vi "7961 FPGA.vi"() -> ()   [LabVIEW 2015]
uses:
  Controls/FPGA_Frame State.ctl
  <vilib>/Platform/TimedLoop/XDataNode/timing_clust.ctl
  <vilib>/Platform/TimedLoop/XDataNode/nitl_modes.ctl
  <vilib>/Platform/TimedLoop/XDataNode/wakeup.ctl
  <vilib>/rvi/FXPMathLib/FxpDiv/subVIs/nifxpmath_Div_SimConfig.ctl
  <vilib>/rvi/Emulation/niFpgaSctlEmulationGetInTimedLoop.vi
  <vilib>/rvi/Emulation/niFpgaProcessEmulError.vi
  <vilib>/rvi/Emulation/niFpgaEmulationReportErrorSimple.vi
  <vilib>/rvi/Emulation/niFpgaGetClockAttributes.vi
  <vilib>/rvi/Emulation/niFpgaCriticalErrorInLSC.vi
  <vilib>/rvi/eio/common/nirviEmuTemplateMethod_errors.vi
  <vilib>/rvi/interface/RandomDataEmulation/niFpgaRandomDataHandleErrors.vi
  <vilib>/rvi/Memory/Memory_Emulation/nirvimemoryFastEmulation.vi
  <vilib>/rvi/Memory/Memory_Emulation/nirvimemoryEmulation.vi
  <vilib>/rvi/Emulation/niFpgaEmulationIsFPGAContextNoSignature.vi
  <vilib>/rvi/DataTransferAndStorage/Container/Common/niFpgaContainerGetUniqueNameForEmu.vi
  <vilib>/rvi/errors/nirviReportUnexpectedCaseInternalError (U32).vi
  <vilib>/rvi/FXPMathLib/FxpDiv/simVIs/DllFxpDivTemp_sub.vi
  <vilib>/Platform/TimedLoop/XDataNode/XDataNode.xnode
  <vilib>/eio/EIONode/EIONode.xnode
  <vilib>/rvi/DataTransferAndStorage/Container/XNode/niFpgaContainer.xnode
  <vilib>/rvi/interface/RandomDataEmulation/nirviRandomDataFpgaReadWriteTemplate.vi
  <vilib>/rvi/FXPMathLib/FxpDiv/XNode/nifxpmath_Div.xnode
  <vilib>/Platform/TimedLoop/XDataNode/XDNodeRunTimeDep.lvlib
  <instrlib>/_niInstr/Basic Elements/v1/FPGA/niInstr Basic Elements v1 FPGA.lvlib
panel:
  in  "Remind":u32
  in  "Switch":bool
  in  "Point/Pixel":i16
  out "Ramp Number":u32
  out "Ramp 待读取元素数量":u32
  in  "Microscope":enum16{"Miniature", "Benchtop"}(ring)
  out "No Remind":bool
  out "Remind Element":u32
  in  "FOCUS":bool
  out "Wait Frame State":T1
  in  "Line":u16
  out "输出有效":bool
  out "运算溢出":bool
  in  "Pixel/Line":u16
  in  "Sanple Rate Divider":u16=1 min=1
  out "Adapter Module Present":bool
  out "Adapter Module ID Expected":u32
  out "Adapter Module ID Inserted":u32
  out "Adapter Module Initialization Done":bool
  out "Adapter Module ID Mismatch":bool
  in  "Adapter Module Do User Command Commit":bool caption="(Mech Action: Latch)"
  in  "Adapter Module User Command":u8
  out "Adapter Module User Command Idle":bool
  out "Adapter Module User Command Status":u8
  in  "Adapter Module User Data 0":u8
  in  "Adapter Module User Data 1":u8
  out "Adapter Module PLL Locked":bool
  # "Acquisition Parameters"
  # "Acquisition Control"
  # "User Command Load"
  # "Fpga status"
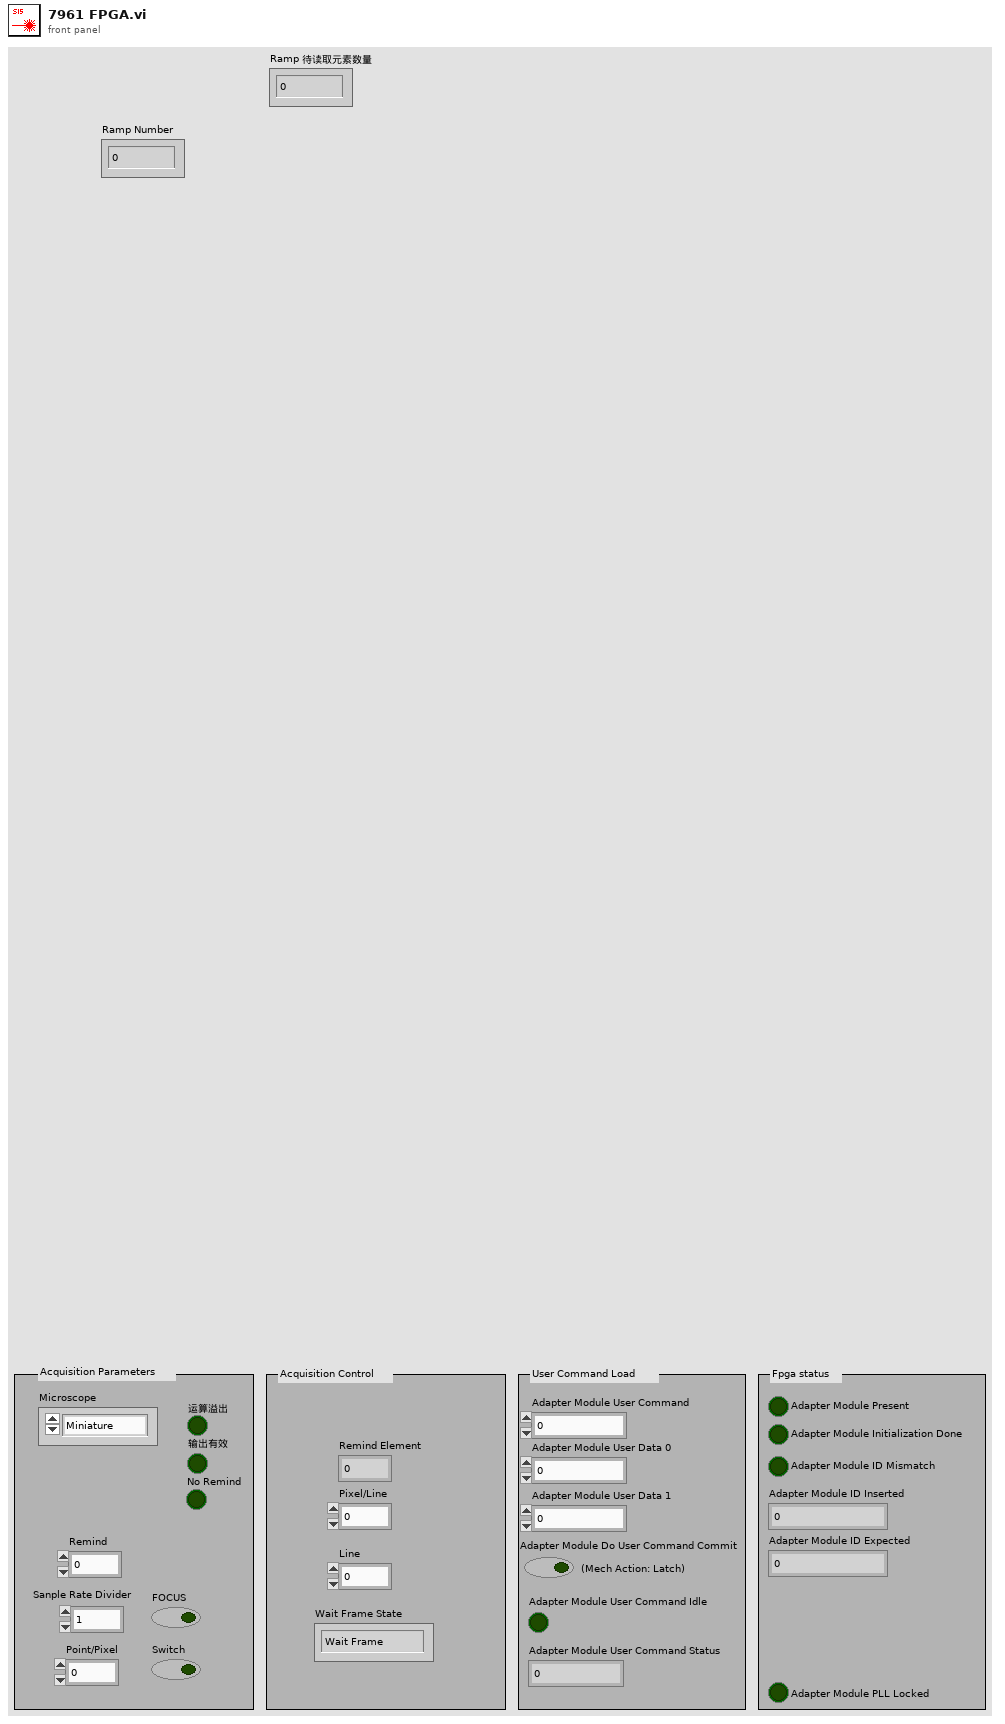
[diagram p1: front panel]
types:
  T1 = typedef "FPGA_Frame State.ctl" = enum16{"Wait Frame", "Start Frame", "Framing"}
  T2 = typedef "XDNodeRunTimeDep.lvlib/timing_clust.ctl" = cluster{"Expected End [f-1]":u64, "Actual End [f-1]":u64, "Finished Late? [f-1]":bool, "Expected End [i-1]":u64, "Actual End [i-1]":u64, "Finished Late? [i-1]":bool, "Expected Start [i]":u64, "Actual Start [i]":u64, "Expected Start [f]":u64, "Actual Start [f]":u64, "Source Name":string, "Structure Name":string, "Period":i64, "Deadline":i64, "Offset":i64, "Start":i64, "Priority":i32, "Timeout":i32, "Mode":T3, "Wakeup Reason":T4, "Error":errorcluster, "Source Type":string, "Secondary Source Type":string, "Global End Time":u64, "Global Start Time":u64, "Frame Duration":u64, "Iteration Duration":u64, "Assigned CPU":i32, "I/O Scan Engine Mode":u32}
  T3 = typedef "XDNodeRunTimeDep.lvlib/nitl_modes.ctl" = enum32{"No Change", "Process missed periods, maintain original phase", "Discard missed periods, maintain original phase", "Process missed periods, ignore original phase", "Discard missed periods, ignore original phase"}
  T4 = typedef "XDNodeRunTimeDep.lvlib/wakeup.ctl" = enum32{"Normal", "Aborted", "Asynchronous wakeup", "Timing source error", "Timed loop error", "Timeout"}
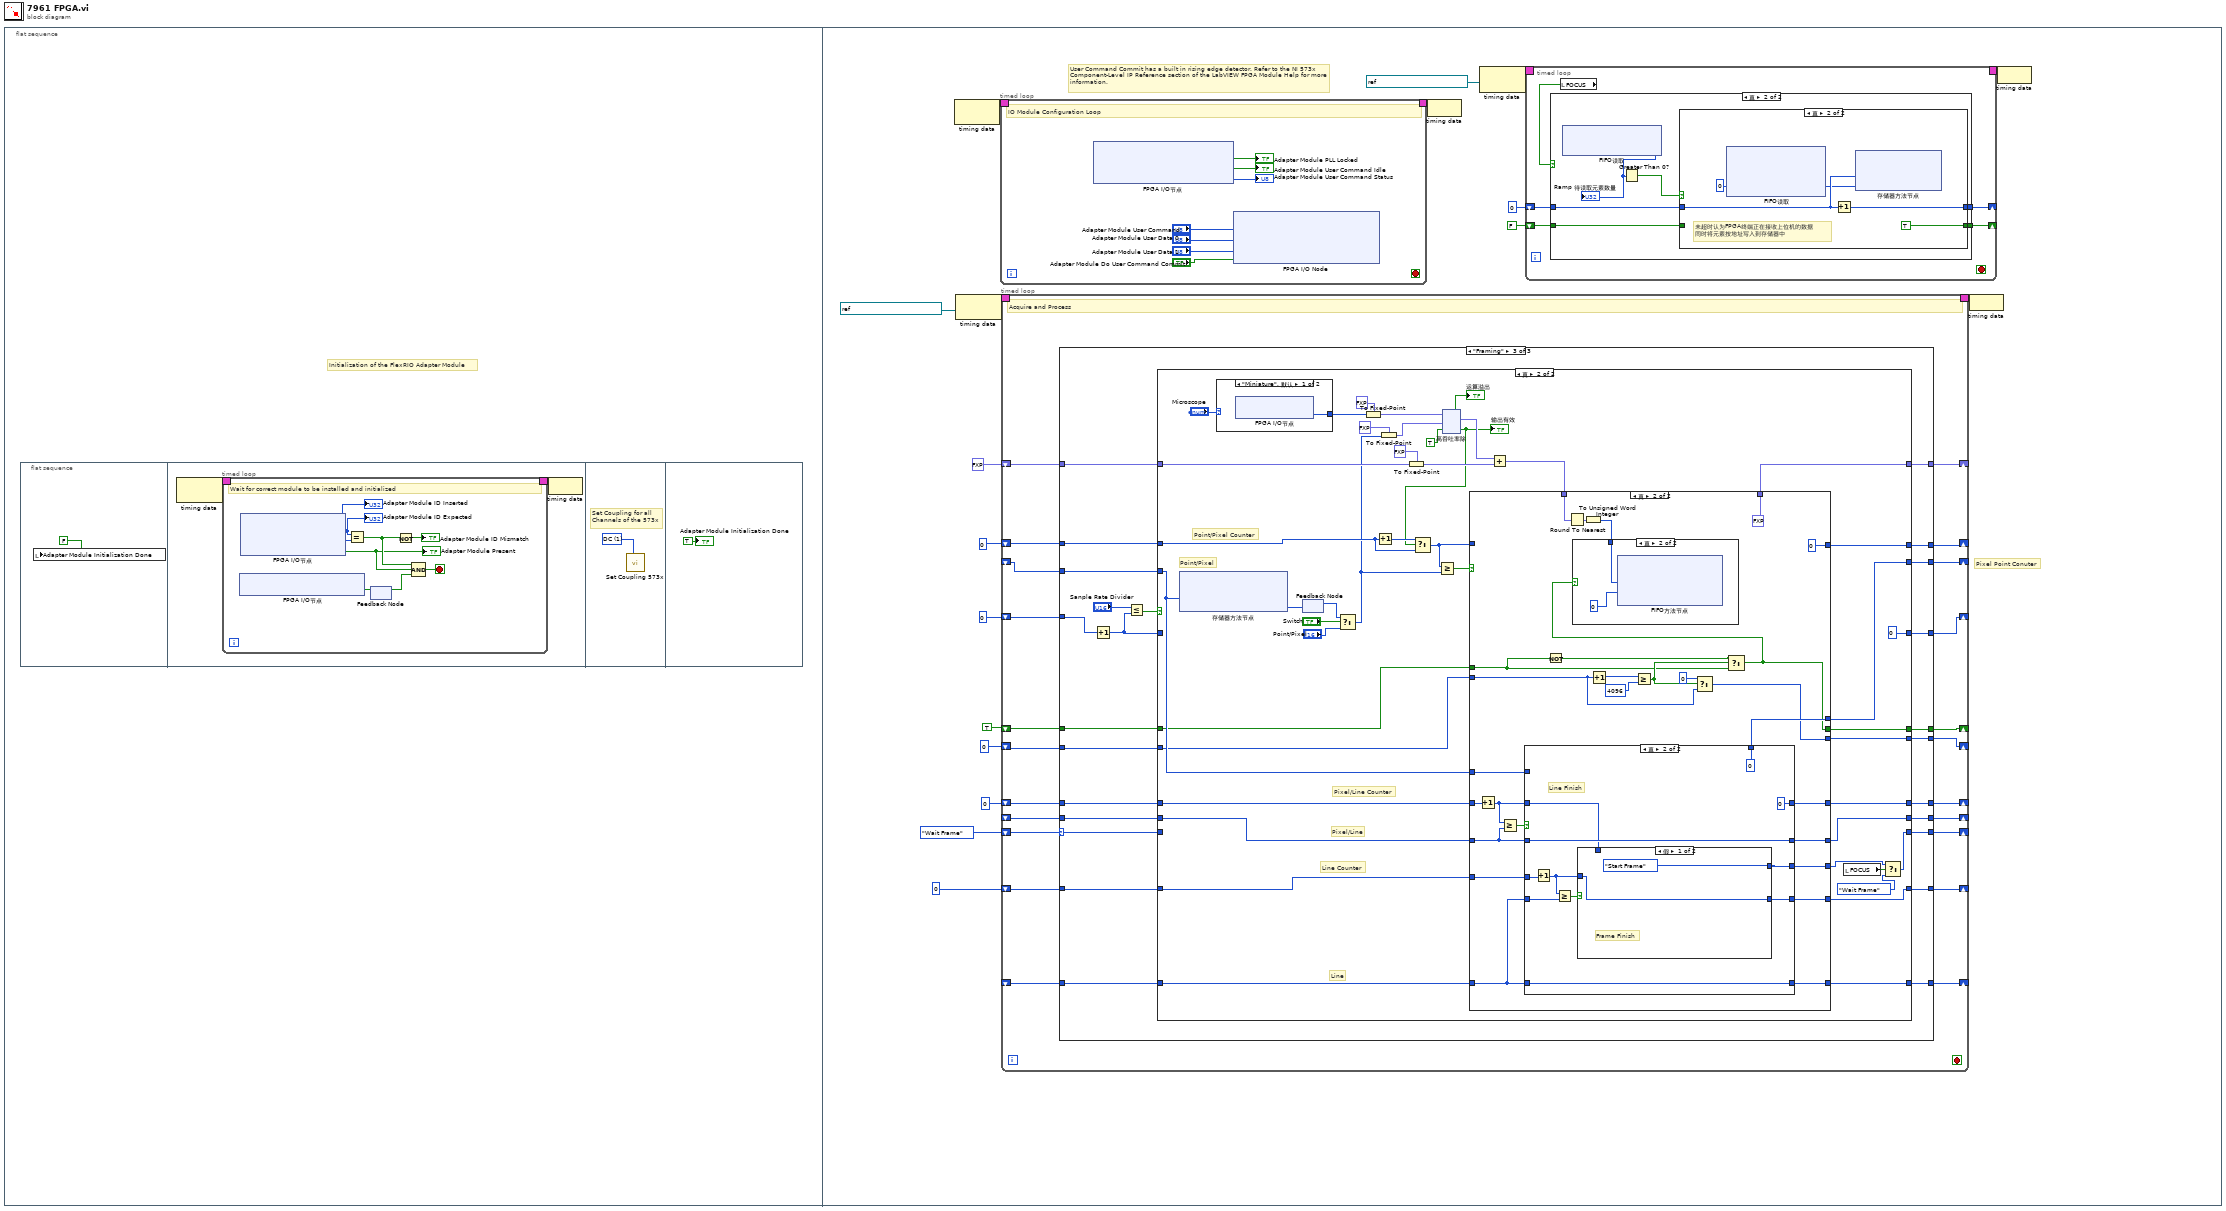
[diagram p0: block diagram]
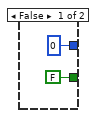
[diagram p2: hidden frame]
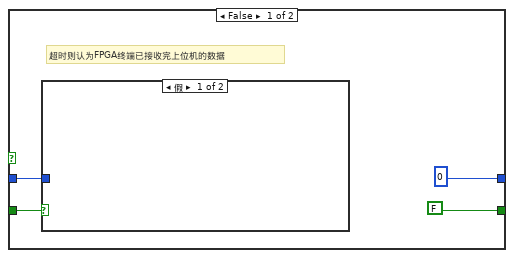
[diagram p3: hidden frame]
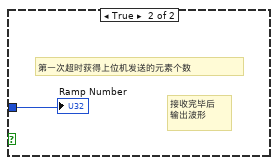
[diagram p4: hidden frame]
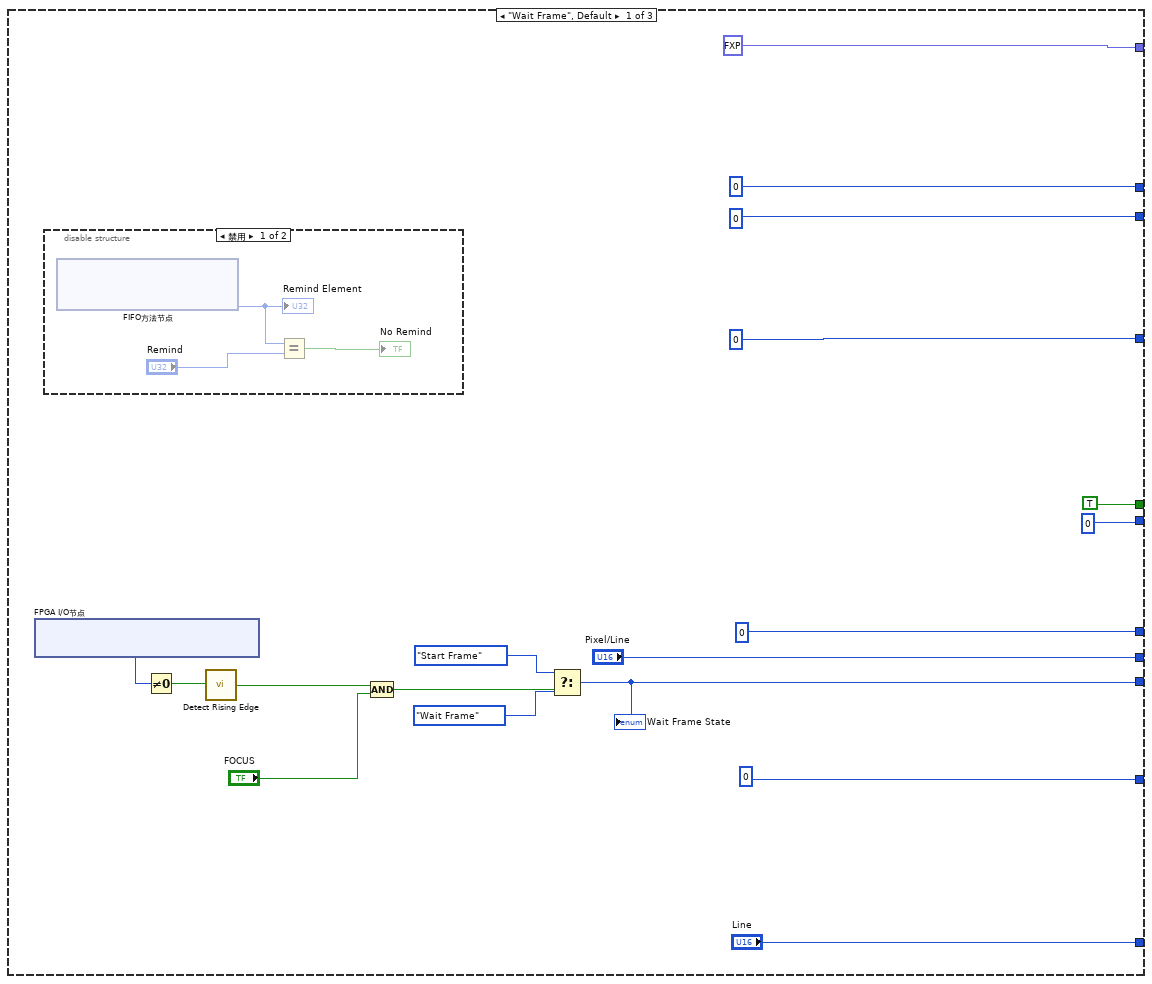
[diagram p5: hidden frame]
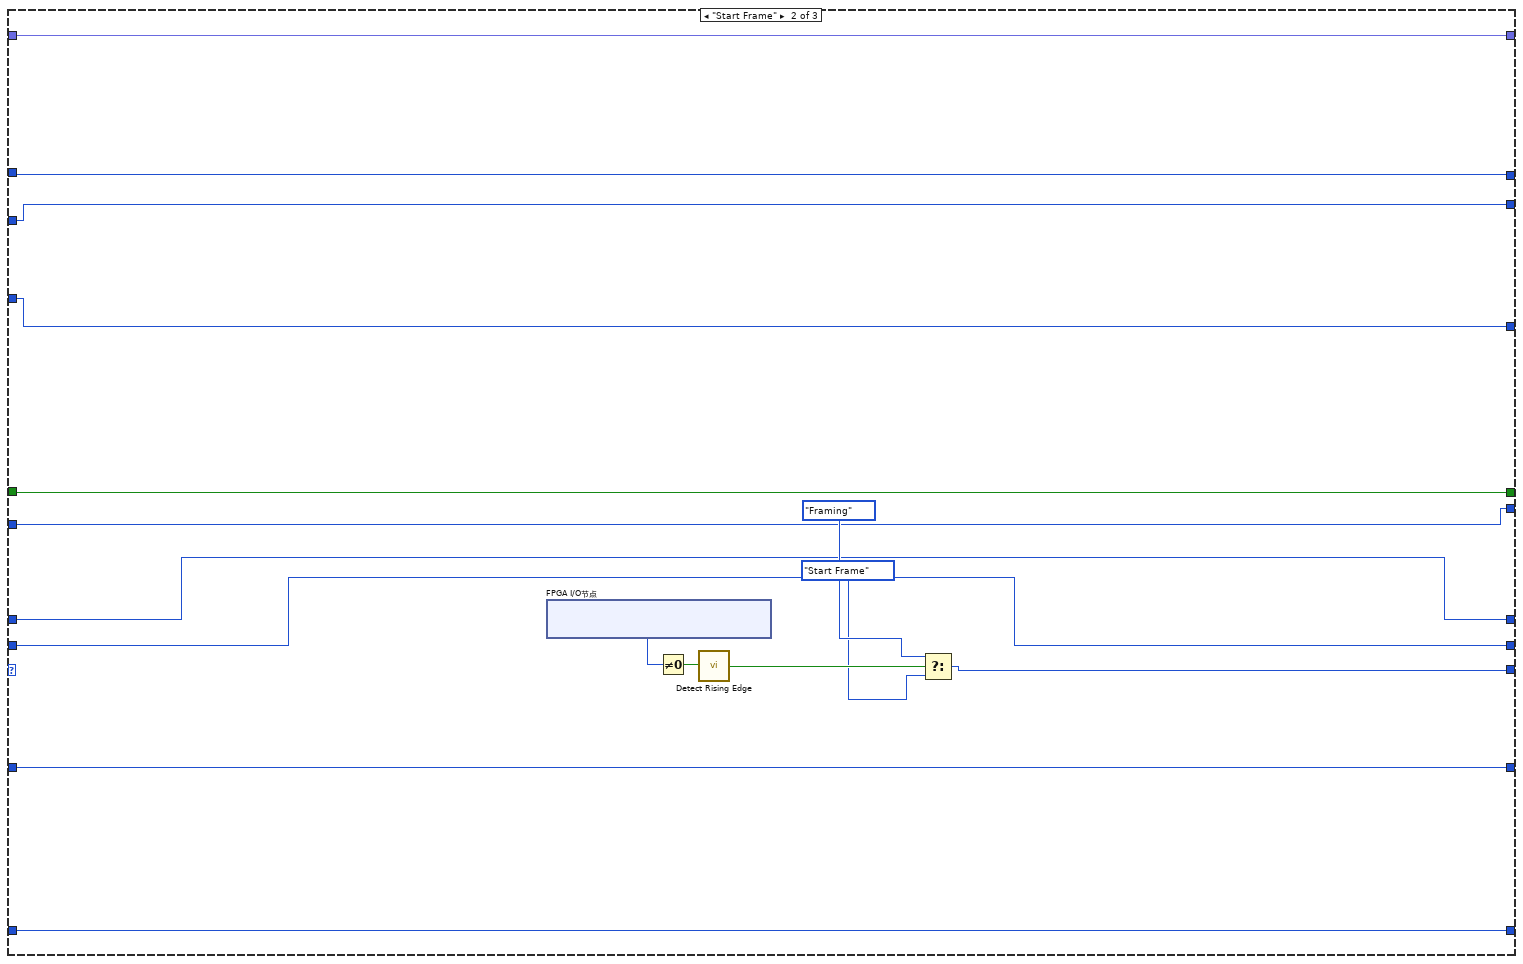
[diagram p7: hidden frame]
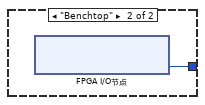
[diagram p9: hidden frame]
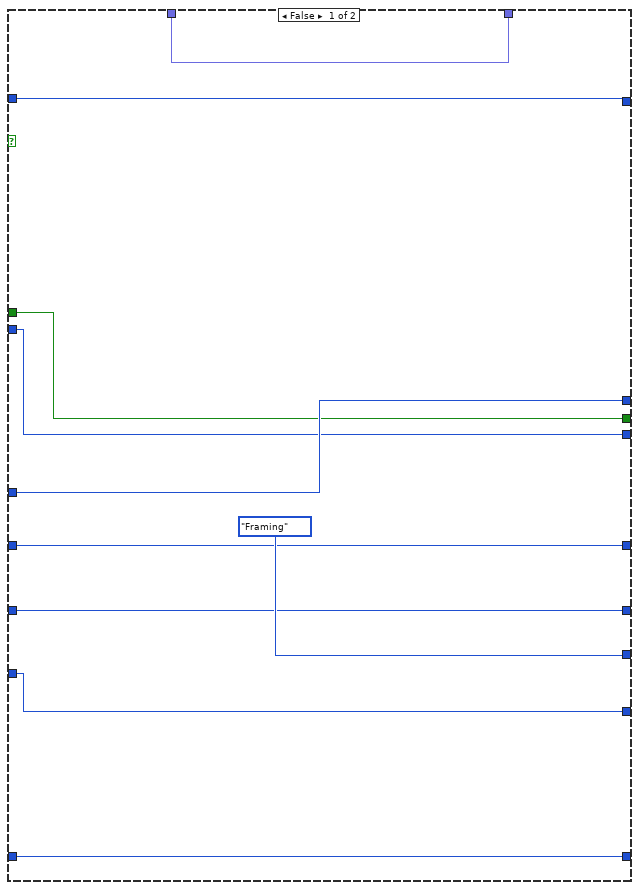
[diagram p10: hidden frame]
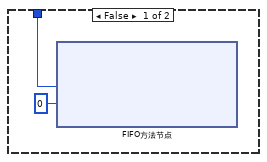
[diagram p11: hidden frame]
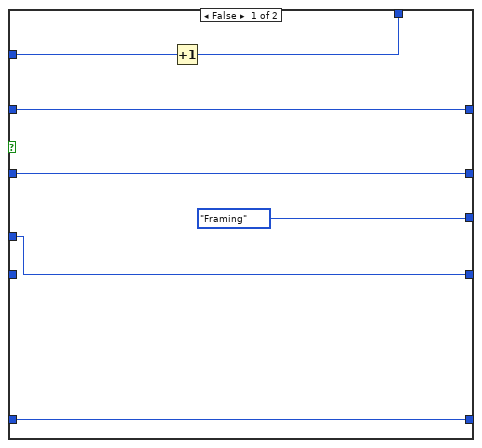
[diagram p12: hidden frame]
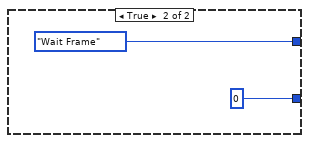
[diagram p13: hidden frame]
diagram:
  n1 = flat-sequence {
    frame #0 {
      # "Initialization of the FlexRIO Adapter Module"
      n2 = flat-sequence {
        frame #0 {
          n3 = local write "Adapter Module Initialization Done"(FALSE ("InitializationDone")) -> ()
        }
        frame #1 {
          n4 = node-c288() -> (w3:T2)  [unwired: 1 in]
          n5 = timed-loop {
            timing: w3 -> [_]
            timing-out: [_] -> w2
            stop <- w10 stop-if-true
            # "Wait for correct module to be installed and initialized"
            n6 = xnode "FPGA I/O节点"() -> ("IO Module\\Initialization Done"=w5:bool)  [unwired: 1 in, 1 out]
            n7 = xnode "FPGA I/O节点"() -> ("Expected IO Module ID"=w11:u32, "Inserted IO Module ID"=w9:u32, "IO Module Present"=w6:bool)  [unwired: 3 in, 3 out]
            "Adapter Module ID Inserted" <- w9
            "Adapter Module ID Expected" <- w11
            "Adapter Module Present" <- w6
            n8 = Equal?(x=w11, y=w9) -> (x = y?=w7:bool)
            n9 = feedback-in #1(w5) -> ()
            n10 = feedback #1() -> (w4:bool)  [unwired: 1 in]
            n11 = Not(x=w7) -> (.not. x?=→"Adapter Module ID Mismatch":bool)
            n12 = Compound Arithmetic op=AND(w7, w6, w4) -> (w10:bool)
          }
          n13 = node-c288(w2) -> ()
        }
        frame #2 {
          w16 = u8 1 items=["DC"=1, "AC"=0] ("Coupling")
          # "Set Coupling for all\nChannels of the 573x"
          n14 = call "Set Coupling 573x.vi"("Coupling"=w16) -> ()  [unwired: 11 in]
        }
        frame #3 {
          "Adapter Module Initialization Done" <- TRUE ("InitializationDone")
        }
      }
    }
    frame #1 {
      # "Pixel Point Conuter"
      # "User Command Commit has a built in rising edge detector. Refer to the NI 573x Component-Level IP Reference section of the LabVIEW FPGA Module Help for more information."
      n15 = node-c288() -> (w35:T2)  [unwired: 1 in]
      n16 = node-c288(refnum<k21> "IO Module\\Sample Clock" ("Source Name")) -> (w33:T2)
      n17 = timed-loop {
        timing: w35 -> [_]
        timing-out: [_] -> w34
        stop <- _ stop-if-true
        # "IO Module Configuration Loop"
        n18 = xnode "FPGA I/O节点"() -> ("IO Module\\PLL Locked"=→"Adapter Module PLL Locked":bool, "IO Module\\User Command Idle"=→"Adapter Module User Command Idle":bool, "IO Module\\User Command Status"=→"Adapter Module User Command Status":u8)  [unwired: 3 in, 3 out]
        n19 = xnode ("FPGA I/O Node")("IO Module\\User Command"="Adapter Module User Command", "IO Module\\User Data 0"="Adapter Module User Data 0", "IO Module\\User Data 1"="Adapter Module User Data 1", "IO Module\\User Command Commit"="Adapter Module Do User Command Commit") -> ()  [unwired: 4 in, 4 out]
      }
      n20 = timed-loop {
        timing: w33 -> [_]
        timing-out: [_] -> w32
        shift-right: [w85] -> _
        shift-left: u16 0 -> [w86]
        shift-right: [w83] -> _
        shift-left: FPGA_Frame_State."Wait Frame" ("Line State") -> [w84]
        shift-right: [w81] -> _
        shift-left: 0 ("t") -> [w82]
        shift-right: [w79] -> _
        shift-left: u16 0 ("t") -> [w80]
        shift-right: [w77] -> _
        shift-left: fxp<+,32,16> 0.0 ("x") -> [w78]
        shift-right: [w75] -> _
        shift-left: u16 0 ("t") -> [w76]
        shift-right: [w73] -> _
        shift-left: _ -> [w74]
        shift-right: [w71] -> _
        shift-left: _ -> [w72]
        shift-right: [w69] -> _
        shift-left: _ -> [w70]
        shift-right: [w67] -> _
        shift-left: TRUE ("x >= y?") -> [w68]
        shift-right: [w65] -> _
        shift-left: u16 0 -> [w66]
        stop <- _ stop-if-true
        # "Acquire and Process"
        n21 = case shown="\"Framing\"" w84 {
          selector: w84 -> [_ _ w146]
          tunnel: w86 -> [_ w112 w148]
          tunnel: [u16 0 w112 w147] -> w85
          tunnel: [w98 w119 w145] -> w83
          tunnel: w82 -> [_ w110 w141]
          tunnel: [0 ("t") w110 w140] -> w81
          tunnel: w80 -> [_ w113 w139]
          tunnel: [u16 0 ("t") w113 w138] -> w79
          tunnel: w78 -> [_ w111 w137]
          tunnel: [fxp<+,32,16> 0.0 ("x") w111 w136] -> w77
          tunnel: w76 -> [_ w121 w135]
          tunnel: [u16 0 ("t") w121 w134] -> w75
          tunnel: w74 -> [_ w116 w133]
          tunnel: [0 ("t") w116 w131] -> w73
          tunnel: w72 -> [_ w115 w132]
          tunnel: ["Pixel/Line" w115 w130] -> w71
          tunnel: w70 -> [_ w114 w129]
          tunnel: ["Line" w114 w128] -> w69
          tunnel: w68 -> [_ w109 w127]
          tunnel: [TRUE ("x >= y?") w109 w126] -> w67
          tunnel: w66 -> [_ w108 w125]
          tunnel: [u16 0 ("t") w108 w124] -> w65
          frame "Wait Frame", Default {
            n22 = xnode "FPGA I/O节点"() -> ("IO Module\\DIO Port 1 Rd Data"=w101:u8)  [unwired: 1 in, 1 out]
            n23 = disable-structure shown="禁用" {
              frame Disabled {
                n24 = xnode ("FIFO方法节点")() -> ("待写入元素数量"=w107:u32)  [unwired: 1 in, 1 out]
                "Remind Element" <- w107
                n25 = Equal?(x=w107, y="Remind") -> (x = y?=→"No Remind":bool)
              }
              frame Enabled {
              }
            }
            n26 = Not Equal To 0?(x=w101) -> (x != 0?=w102:bool)
            n27 = call <instrlib>:"Detect Rising Edge.vi"("signal"=w102) -> ("edge detected"=w91:bool)  [unwired: 14 in]
            n28 = Compound Arithmetic op=AND(w91, "FOCUS") -> (w90:bool)
            n29 = Select(t=FPGA_Frame_State."Start Frame" ("Line State"), s=w90, f=FPGA_Frame_State."Wait Frame" ("Line State")) -> (s? t:f=w98:T1)
            "Wait Frame State" <- w98
          }
          frame "Start Frame" {
            n30 = xnode "FPGA I/O节点"() -> ("IO Module\\DIO Port 0 Rd Data"=w122:u8)  [unwired: 1 in, 1 out]
            n31 = Not Equal To 0?(x=w122) -> (x != 0?=w123:bool)
            n32 = call <instrlib>:"Detect Rising Edge.vi"("signal"=w123) -> ("edge detected"=w120:bool)  [unwired: 14 in]
            n33 = Select(t=FPGA_Frame_State."Framing" ("Line State"), s=w120, f=FPGA_Frame_State."Start Frame" ("Line State")) -> (s? t:f=w119:T1)
          }
          frame "Framing" {
            n34 = Increment(x=w148) -> (x+1=w144:u16)
            n35 = Less Or Equal?(x="Sanple Rate Divider", y=w144) -> (x <= y?=w142:bool)
            n36 = case shown="真" w142 {
              tunnel: [w159 u16 0] -> w147
              tunnel: w144 -> [w159 _]
              tunnel: w146 -> [w158 _]
              tunnel: [w158 w181] -> w145
              tunnel: w141 -> [w157 w175]
              tunnel: [w157 w196] -> w140
              tunnel: w139 -> [w156 w182]
              tunnel: [w156 w188] -> w138
              tunnel: w137 -> [w155 w201]
              tunnel: [w155 w197] -> w136
              tunnel: w135 -> [w154 w190]
              tunnel: [w154 w189] -> w134
              tunnel: w133 -> [w153 w172]
              tunnel: w132 -> [w152 w185]
              tunnel: [w153 w173] -> w131
              tunnel: [w152 w186] -> w130
              tunnel: w129 -> [w151 w187]
              tunnel: [w151 w183] -> w128
              tunnel: w127 -> [w150 w161]
              tunnel: [w150 w163] -> w126
              tunnel: w125 -> [w149 w160]
              tunnel: [w149 w162] -> w124
              frame False {
              }
              frame True {
                # "Point/Pixel"
                # "Line Counter"
                # "Line"
                # "Point/Pixel Counter"
                # "Pixel/Line Counter"
                # "Pixel/Line"
                n37 = xnode ("存储器方法节点")("地址"=w172) -> ("数据"=w168:i16)  [unwired: 1 in, 1 out]
                n38 = case shown="\"Miniature\", 默认" "Microscope" {
                  tunnel: [w204 w205] -> w195
                  frame "Miniature", Default {
                    n39 = xnode "FPGA I/O节点"() -> ("IO Module\\AI 0"=w204:u16)  [unwired: 1 in, 1 out]
                  }
                  frame "Benchtop" {
                    n40 = xnode "FPGA I/O节点"() -> ("IO Module\\AI 1"=w205:u16)  [unwired: 1 in, 1 out]
                  }
                }
                n41 = feedback-in #2(w168) -> ()
                n42 = feedback #2 ("反馈节点")() -> (w167:i16)  [unwired: 1 in]
                n43 = Select(t=w167, s="Switch", f="Point/Pixel") -> (s? t:f=w166:i16)
                n44 = To Fixed-Point(fixed-point type=fxp<+,32,16> 0.0 ("x"), number=w195) -> (fixed-point=w194:fxp<+,32,16>)
                n45 = Increment(x=w175) -> (x+1=w176:i32)
                n46 = To Fixed-Point(fixed-point type=fxp<+,32,16> 0.0 ("x"), number=w166) -> (fixed-point=w191:fxp<+,32,16>)
                n47 = To Fixed-Point(fixed-point type=fxp<+,32,16> 0.0 ("x"), number=w201) -> (fixed-point=w171:fxp<+,32,16>)
                n48 = xnode "高吞吐率除"("x"=w194, "y"=w191, "输入有效"=TRUE) -> ("x/y"=w200:fxp<+,32,16>, "运算溢出"=→"运算溢出":bool, "输出有效"=w169:bool)  [unwired: 1 in, 1 out]
                "输出有效" <- w169
                n49 = Select(t=w176, s=w169, f=w175) -> (s? t:f=w177:i32)
                n50 = Greater Or Equal?(x=w177, y=w166) -> (x >= y?=w184:bool)
                n51 = Add(x=w200, y=w171) -> (x+y=w198:fxp<+,33,17>)
                n52 = case shown="真" w184 {
                  tunnel: w198 -> [w214 w227]
                  tunnel: [w214 fxp<+,32,16> 0.0 ("x")] -> w197
                  tunnel: [w215 0 ("t")] -> w196
                  tunnel: w177 -> [w215 _]
                  tunnel: w182 -> [w210 w234]
                  tunnel: w190 -> [w209 w240]
                  tunnel: [w209 w239] -> w189
                  tunnel: [FPGA_Frame_State."Framing" ("Line State") w238] -> w179
                  tunnel: [w210 w233] -> w188
                  tunnel: w187 -> [w212 w236]
                  tunnel: [w211 w235] -> w186
                  tunnel: w185 -> [w211 w231]
                  tunnel: [w212 w237] -> w183
                  tunnel: [w208 w228] -> w173
                  tunnel: w172 -> [w208 w229]
                  tunnel: [w206 w219] -> w163
                  tunnel: [w207 w216] -> w162
                  tunnel: w161 -> [w206 w218]
                  tunnel: w160 -> [w207 w217]
                  frame False {
                  }
                  frame True {
                    n53 = Increment(x=w234) -> (x+1=w232:u16)
                    n54 = Greater Or Equal?(x=w232, y=w231) -> (x >= y?=w230:bool)
                    n55 = case shown="真" w230 {
                      tunnel: w240 -> [w249 w264]
                      tunnel: [w249 w263] -> w239
                      tunnel: [FPGA_Frame_State."Framing" ("Line State") w262] -> w238
                      tunnel: w236 -> [_ w259]
                      tunnel: [w253 w258] -> w237
                      tunnel: w236 -> [w253 w258]
                      tunnel: [w252 w257] -> w235
                      tunnel: w231 -> [w252 w257]
                      tunnel: [w251 u16 0] -> w233
                      tunnel: w232 -> [w251 w255]
                      tunnel: w229 -> [w248 _]
                      tunnel: [w247 0] -> w228
                      frame False {
                        n56 = Increment(x=w248) -> (x+1=w247:i32)
                      }
                      frame True {
                        # "Line Finish"
                        n57 = Increment(x=w264) -> (x+1=w260:u16)
                        n58 = Greater Or Equal?(x=w260, y=w259) -> (x >= y?=w261:bool)
                        n59 = case shown="假" w261 {
                          tunnel: w260 -> [w265 _]
                          tunnel: [w265 u16 0] -> w263
                          tunnel: [FPGA_Frame_State."Start Frame" ("Line State") FPGA_Frame_State."Wait Frame" ("Line State")] -> w262
                          tunnel: w255 -> [_ _]
                          frame False {
                            # "Frame Finish"
                          }
                          frame True {
                          }
                        }
                      }
                    }
                    n60 = Not(x=w218) -> (.not. x?=w221:bool)
                    n61 = Round To Nearest(number=w227) -> (nearest integer value=w225:fxp<+,18,18>)
                    n62 = To Unsigned Word Integer(number=w225) -> (unsigned 16bit integer=w226:u16)
                    n63 = Increment(x=w217) -> (x+1=w220:u16)
                    n64 = Greater Or Equal?(x=w220, y=u16 4096) -> (x >= y?=w223:bool)
                    n65 = Select(t=u16 0, s=w223, f=w217) -> (s? t:f=w216:u16)
                    n66 = Select(t=w221, s=w223, f=w218) -> (s? t:f=w219:bool)
                    n67 = case shown="真" w219 {
                      tunnel: w226 -> [w244 w245]
                      frame False {
                        n68 = xnode ("FIFO方法节点")("元素"=w244, "超时"=0) -> ()  [unwired: 1 in, 2 out]
                      }
                      frame True {
                        n69 = xnode ("FIFO方法节点")("元素"=w245, "超时"=0) -> ()  [unwired: 1 in, 2 out]
                      }
                    }
                  }
                }
                n70 = local read "FOCUS"() -> (w180:bool)
                n71 = Select(t=w179, s=w180, f=FPGA_Frame_State."Wait Frame" ("Line State")) -> (s? t:f=w181:T1)
              }
            }
          }
        }
      }
      n72 = node-c288(w34) -> ()
      n73 = node-c288(refnum<k21> "IO Module\\Sample Clock" ("Source Name")) -> (w25:T2)
      n74 = timed-loop {
        shift-right: [w39] -> _
        shift-left: u32 0 ("地址") -> [w40]
        shift-right: [w37] -> _
        shift-left: FALSE ("执行") -> [w38]
        timing: w25 -> [_]
        timing-out: [_] -> w24
        stop <- _ stop-if-true
        n75 = local read "FOCUS"() -> (w36:bool)
        n76 = case shown="真" w36 {
          tunnel: w40 -> [_ w48]
          tunnel: [u32 0 w47] -> w39
          tunnel: w38 -> [_ w46]
          tunnel: [FALSE w45] -> w37
          frame False {
          }
          frame True {
            n77 = xnode ("FIFO读取")() -> ("待读取元素数量"=w43:u32)  [unwired: 1 in, 1 out]
            "Ramp 待读取元素数量" <- w43
            n78 = Greater Than 0?(x=w43) -> (x > 0?=w44:bool)
            n79 = case shown="真" w44 {
              tunnel: w48 -> [w50 w57]
              tunnel: [u32 0 w56] -> w47
              tunnel: w46 -> [w51 _]
              tunnel: [FALSE TRUE] -> w45
              frame False {
                # "超时则认为FPGA终端已接收完上位机的数据"
                n80 = case shown="假" w51 {
                  tunnel: w50 -> [_ w53]
                  frame False {
                  }
                  frame True {
                    # "接收完毕后\n输出波形"
                    # "第一次超时获得上位机发送的元素个数"
                    "Ramp Number" <- w53
                  }
                }
              }
              frame True {
                # "未超时认为FPGA终端正在接收上位机的数据\n同时将元素按地址写入到存储器中"
                n81 = xnode ("FIFO读取")("超时"=0) -> ("元素"=w54:i16)  [unwired: 1 in, 2 out]
                n82 = Increment(x=w57) -> (x+1=w56:u32)
                n83 = xnode ("存储器方法节点")("地址"=w57, "数据"=w54) -> ()  [unwired: 1 in, 1 out]
              }
            }
          }
        }
      }
      n84 = node-c288(w32) -> ()
      n85 = node-c288(w24) -> ()
    }
  }
